vi "Destroy User Events - ExitMultiLoop.vi"(8 "error in (no error)":errorcluster, 10 "user event array":refnum<user-event>[](array[refnum])) -> (0 "error out":errorcluster)   [LabVIEW 2018, in "UserEvent-ExitEventLoop.lvlib"]
doc: "Destroy the user event, even if there is an incoming error.\n\nBolder Software LLC"
uses:
  UserEvent-ExitEventLoop.lvlib
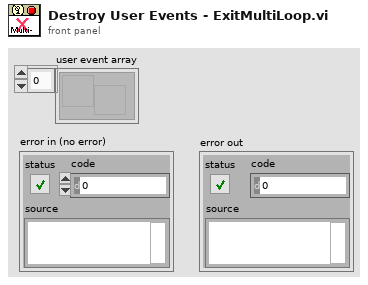
[diagram p1: front panel]
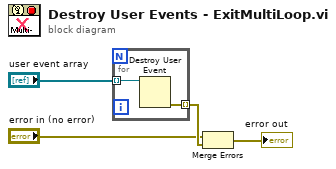
[diagram p0: block diagram]
diagram:
  n1 = for {
    tunnel: [w6] -> w4 mode=indexing
    tunnel: "user event array" -> [w5] mode=indexing
    n2 = Destroy User Event(user event=w5) -> (error out=w6:errorcluster)  [unwired: 1 in]
  }
  n3 = Merge Errors("error in (no error)", w4) -> (→"error out":errorcluster)
